vi "CalculateFpgaTachBuffer.vi"(9 "fpga tach buffer minimum":i32, 10 "fpga tach buffer multiplier":i32, 11 "pulses per rev":i32[](array[numeric])) -> (3 "Fpga Tach Buffer Size (samples)":i32)   [LabVIEW 2017, in "CmsAcquisition.lvlib"]
uses:
  <vilib>/addons/InsightCM/Devices/Shared/Cms/CmsAcquisition/CmsAcquisition.lvlib
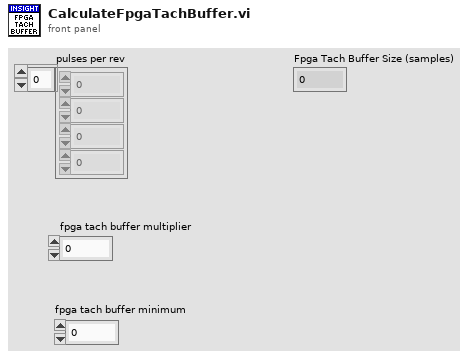
[diagram p1: front panel]
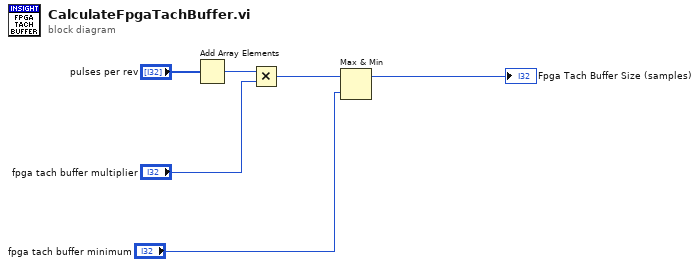
[diagram p0: block diagram]
diagram:
  n1 = Add Array Elements(numeric array="pulses per rev") -> (sum=w5:i32)
  n2 = Multiply(x=w5, y="fpga tach buffer multiplier") -> (x*y=w3:i32)
  n3 = Max & Min(x=w3, y="fpga tach buffer minimum") -> (max(x,y)=→"Fpga Tach Buffer Size (samples)":i32)  [unwired: 1 out]
